vi "Test Coord Transform.vi"() -> ()   [LabVIEW 2011]
uses:
  gVision.lvlib
panel:
  out "error out":errorcluster
  in  "orientation":cluster{"pitch":dbl, "roll":dbl, "yaw":dbl}
  out "global_out":cluster{"x":dbl, "y":dbl, "z":dbl}
  out "local_out":cluster{"x":dbl, "y":dbl, "z":dbl}
  in  "offset":cluster{"x":dbl, "y":dbl, "z":dbl}
  in  "local_in":cluster{"x":dbl, "y":dbl, "z":dbl}
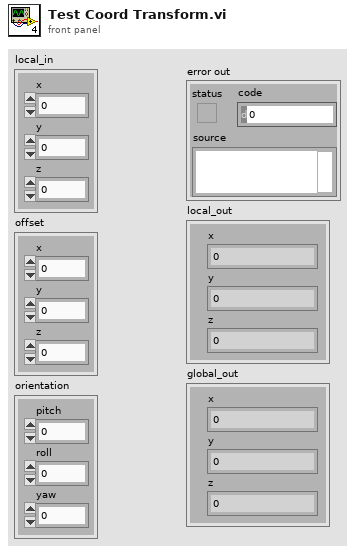
[diagram p1: front panel]
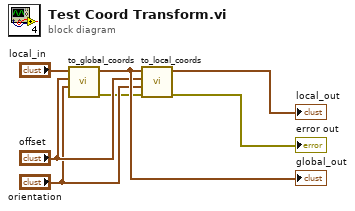
[diagram p0: block diagram]
diagram:
  n1 = call "to_global_coords.vi"("orientation"="orientation", "offset"="offset", "local"="local_in") -> ("error out"=w3:errorcluster, "global"=w6:cluster{"x":dbl, "y":dbl, "z":dbl})  [unwired: 7 in]
  "global_out" <- w6
  n2 = call "to_local_coords.vi"("error in"=w3, "orientation"="orientation", "offset"="offset", "global"=w6) -> ("error out"=→"error out":errorcluster, "local"=→"local_out":cluster{"x":dbl, "y":dbl, "z":dbl})  [unwired: 6 in]
